vi "Handle Last Ack Core.vi"(4 "error in (no error)":errorcluster, 6 "Last Ack":refnum<class "Last Ack.lvclass">, 7 "Chat Room Model in":refnum<class "Chat Window Model.lvclass">) -> (0 "error out":errorcluster, 3 "Chat Room Model out":refnum<class "Chat Window Model.lvclass">)   [LabVIEW 2020, in "Chat Window Model.lvlib" / "Chat Window Model.lvclass"]
doc: "(<B>Filename</B>: Actor Framework.lvlib:Actor.lvclass:Handle Last Ack Core.vi)\n\nDefines how the caller actor responds to the Last Ack message from a nested actor. The Last Ack message is the final message a nested actor sends to its caller before it shuts down. The message contains information about the final state of the nested actor.\n\nBy default, this method does nothing except return any error the nested actor sent. A descendant class may override this method to define behavior."
uses:
  Chat Window Model.lvclass
  <vilib>/ActorFramework/LastAck/Last Ack.lvclass
  C:/Program Files (x86)/National Instruments/LabVIEW 2020/vi.lib/ActorFramework/Actor/Actor.lvclass
  <vilib>/ActorFramework/Actor/Actor.lvclass/Actor.ctl
  <vilib>/ActorFramework/Message Enqueuer/Message Enqueuer.lvclass/Message Enqueuer.ctl
  <vilib>/ActorFramework/Message Enqueuer/Init from Existing Queue.vi
  <vilib>/ActorFramework/Message Enqueuer/Enqueue.vi
  <vilib>/ActorFramework/Stop Msg/Stop Msg.lvclass
  C:/Program Files (x86)/National Instruments/LabVIEW 2020/vi.lib/ActorFramework/Message/Message.lvclass
  <vilib>/ActorFramework/Message Priority Queue/Priority Enqueue.vi
  <vilib>/ActorFramework/Actor/Actor.lvclass
  <vilib>/ActorFramework/Message Enqueuer/Message Enqueuer.lvclass
  Chat Window Model.lvclass/Chat Window Model.ctl
  F:/Gitlab Repository/LabVIEW-Study/10.Top 5 Actor Framework Overrides/Yang's Solution/Chat Room Model/Chat Room Model/Chat Window Model.lvclass
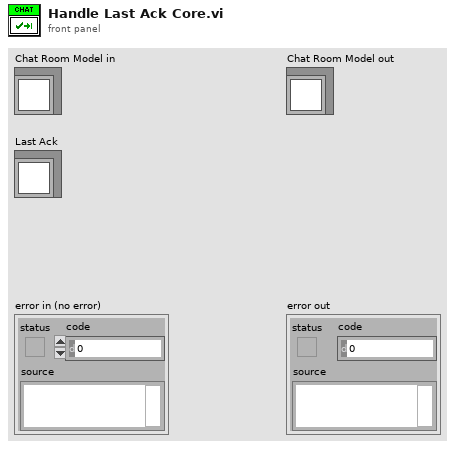
[diagram p1: front panel]
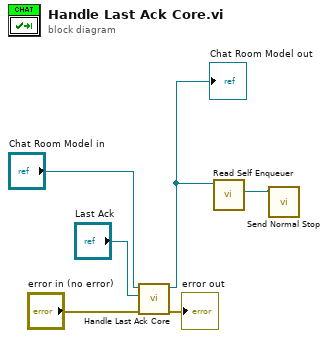
[diagram p0: block diagram]
diagram:
  n1 = call-parent "Handle Last Ack Core.vi"("error in (no error)"="error in (no error)", "Last Ack"="Last Ack", "Actor in"="Chat Room Model in") -> ("error out"=→"error out":errorcluster, "Actor out"=w2:refnum<class "Chat Window Model.lvclass">)  [unwired: 3 in]
  "Chat Room Model out" <- w2
  n2 = call <vilib>:"Read Self Enqueuer.vi"("Actor"=w2) -> ("Self Enqueuer"=w1:refnum<class "Message Enqueuer.lvclass">)  [unwired: 10 in]
  n3 = call <vilib>:"Send Normal Stop.vi"("Message Enqueuer"=w1) -> ()  [unwired: 10 in, 1 out]
